vi "Blink_SDK_example_NoODP.vi"() -> ()   [LabVIEW 2010]
uses:
  Program Files/Meadowlark Optics/Blink OverDrive Plus/SDK/Blink_C_wrapper.dll
panel:
  out "ImgData 2":u8[](array[numeric])
  in  "Wait Timer":dbl
  out "Use External Triggers":bool
  out "Wavefront Correction Path":path
  out "BoardNum":i32
  out "ImgData":u8[](array[numeric])
  # "PCIe  LabVIEWSDK"
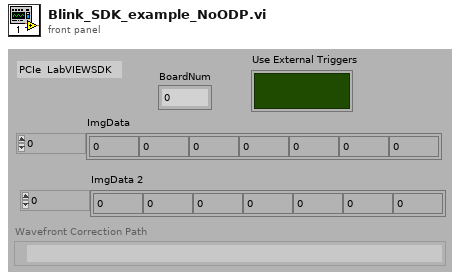
[diagram p1: front panel]
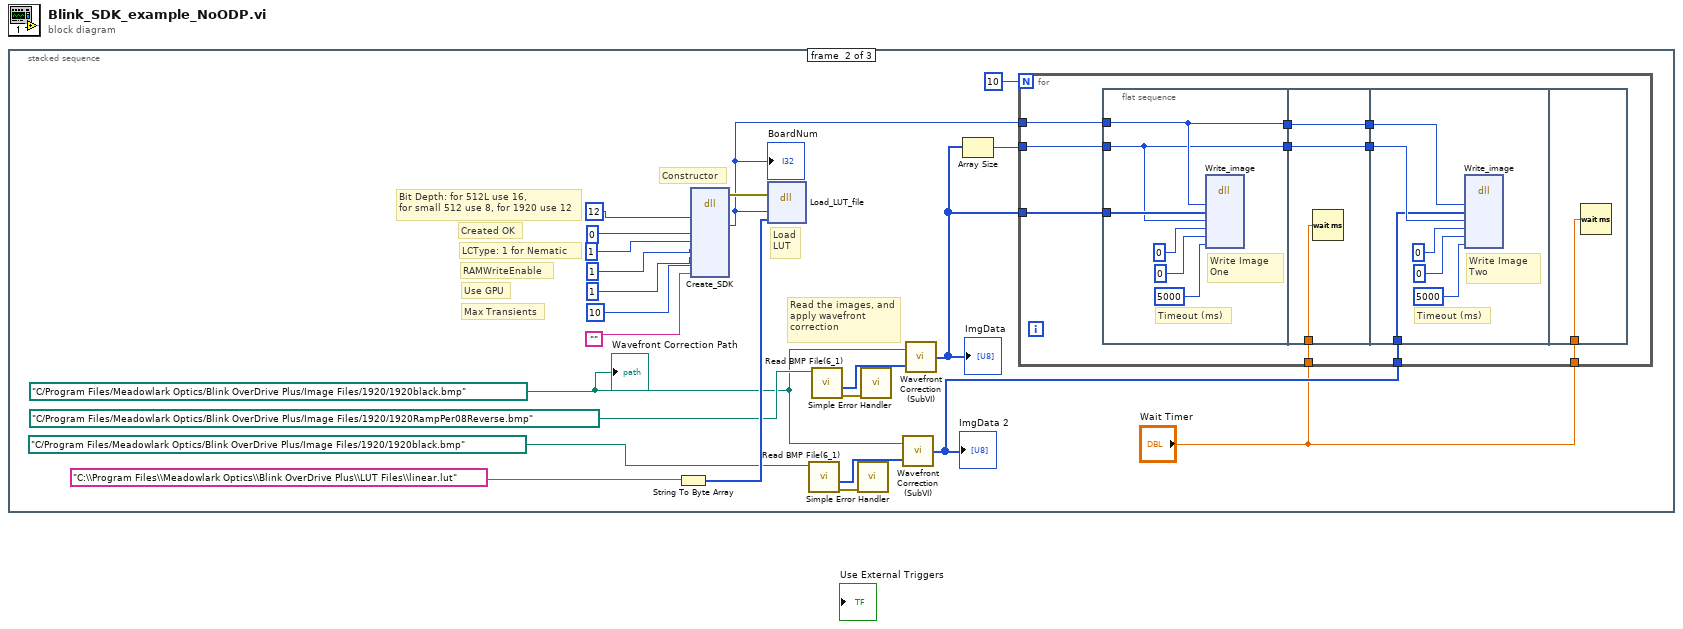
[diagram p0: block diagram]
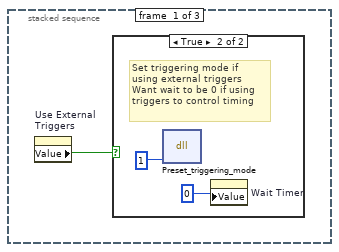
[diagram p2: hidden frame]
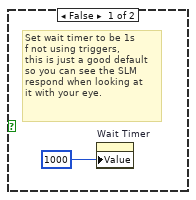
[diagram p3: hidden frame]
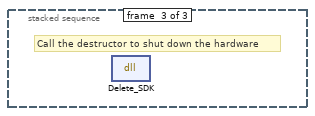
[diagram p4: hidden frame]
diagram:
  n1 = stacked-sequence {
    frame #0 {
      n2 = property on="Use External \nTriggers" class="Bool (strict)"() -> ("Value"=w1:bool)  [unwired: 2 in, 2 out]
      n3 = case shown="True" w1 {
        frame False {
          # "Set wait timer to be 1s \nf not using triggers,\nthis is just a good default \nso you can see the SLM \nrespond when looking at \nit with your eye."
          n4 = property on="Wait Timer" class="DigNum (strict)"("Value"=1000) -> ()  [unwired: 2 in, 2 out]
        }
        frame True {
          # "Set triggering mode if \nusing external triggers\nWant wait to be 0 if using \ntriggers to control timing"
          n5 = dll-call lib="C:/Program Files/Meadowlark Optics/Blink OverDrive Plus/SDK/Blink_C_wrapper.dll" fn="Preset_triggering_mode"("UseTrigger"=1) -> ()  [unwired: 5 in, 2 out]
          n6 = property on="Wait Timer" class="DigNum (strict)"("Value"=0) -> ()  [unwired: 2 in, 2 out]
        }
      }
    }
    frame #1 {
      w10 = path "C:/Program Files/Meadowlark Optics/Blink OverDrive Plus/Image Files/1920/1920black.bmp"
      # "Load\nLUT"
      # "Read the images, and apply wavefront\ncorrection"
      # "Created OK"
      # "Max Transients"
      # "Use GPU"
      # "RAMWriteEnable"
      # "Bit Depth: for 512L use 16, \nfor small 512 use 8, for 1920 use 12"
      # "LCType: 1 for Nematic"
      # "Constructor"
      n7 = String To Byte Array(string="C:\\Program Files\\Meadowlark Optics\\Blink OverDrive Plus\\LUT Files\\linear.lut") -> (unsigned byte array=w21:u8[])
      n8 = dll-call lib="C:/Program Files/Meadowlark Optics/Blink OverDrive Plus/SDK/Blink_C_wrapper.dll" fn="Create_SDK"("SLM_bit_depth"=12, "constructed_ok"=0, "is_nematic_type"=1, "RAM_write_enable"=1, "use_GPU_if_available"=1, "max_transient_frames"=10, "static_regional_lut_file"="") -> (error out=w22:errorcluster, "n_boards_found"=w6:u64)  [unwired: 12 in, 1 out]
      "BoardNum" <- w6
      n9 = dll-call lib="C:/Program Files/Meadowlark Optics/Blink OverDrive Plus/SDK/Blink_C_wrapper.dll" fn="Load_LUT_file"(error in=w22, "Board"=w6, "LUTPath"=w21) -> ()  [unwired: 5 in, 2 out]
      n10 = call <vilib>:"Read BMP File(6_1).vi"("path to BMP file"=path "C:/Program Files/Meadowlark Optics/Blink OverDrive Plus/Image Files/1920/1920black.bmp") -> ("error out"=w17:errorcluster, "flattened image data"=w18:u8[])  [unwired: 5 in, 4 out]
      n11 = call <vilib>:"Read BMP File(6_1).vi"("path to BMP file"=path "C:/Program Files/Meadowlark Optics/Blink OverDrive Plus/Image Files/1920/1920RampPer08Reverse.bmp") -> ("error out"=w19:errorcluster, "flattened image data"=w20:u8[])  [unwired: 5 in, 4 out]
      n12 = call <vilib>:"Simple Error Handler.vi"("error in (no error)"=w17) -> ()  [unwired: 4 in, 5 out]
      n13 = call <vilib>:"Simple Error Handler.vi"("error in (no error)"=w19) -> ()  [unwired: 4 in, 5 out]
      n14 = call "Wavefront Correction (SubVI).vi"("Source Image Array"=w18, "Correction Path"=w10) -> ("Corrected Image Array"=w11:u8[])
      "ImgData 2" <- w11
      n15 = call "Wavefront Correction (SubVI).vi"("Source Image Array"=w20, "Correction Path"=w10) -> ("Corrected Image Array"=w13:u8[])
      "ImgData" <- w13
      n16 = Array Size(array=w13) -> (size(s)=w12:i32)
      n17 = for {
        N: 10 -> [_]
        tunnel: w6 -> [w37]
        tunnel: w13 -> [w36]
        tunnel: w12 -> [w35]
        tunnel: w11 -> [w34]
        tunnel: "Wait Timer" -> [w29]
        tunnel: "Wait Timer" -> [w28]
        n18 = flat-sequence {
          tunnel: w37 -> [w39]
          tunnel: w36 -> [w40]
          tunnel: w35 -> [w38]
          tunnel: [w39] -> w33
          tunnel: [w38] -> w31
          tunnel: w33 -> [w46]
          tunnel: [w46] -> w32
          tunnel: w31 -> [w45]
          tunnel: [w45] -> w30
          tunnel: w29 -> [w44]
          tunnel: w32 -> [w49]
          tunnel: w30 -> [w48]
          tunnel: w34 -> [w47]
          tunnel: w28 -> [w53]
          frame #0 {
            # "Timeout (ms)"
            # "Write Image \nOne"
            n19 = dll-call lib="C:/Program Files/Meadowlark Optics/Blink OverDrive Plus/SDK/Blink_C_wrapper.dll" fn="Write_image"("board"=w39, "Image"=w40, "ImageSize"=w38, "WaitForTrigger"=0, "ExternalPulse"=0, "timeout"=5000) -> ()  [unwired: 10 in, 2 out]
          }
          frame #1 {
            n20 = Wait (ms)(milliseconds to wait=w44) -> ()  [unwired: 1 out]
          }
          frame #2 {
            # "Timeout (ms)"
            # "Write Image \nTwo"
            n21 = dll-call lib="C:/Program Files/Meadowlark Optics/Blink OverDrive Plus/SDK/Blink_C_wrapper.dll" fn="Write_image"("board"=w49, "Image"=w47, "ImageSize"=w48, "WaitForTrigger"=0, "ExternalPulse"=0, "timeout"=5000) -> ()  [unwired: 10 in, 2 out]
          }
          frame #3 {
            n22 = Wait (ms)(milliseconds to wait=w53) -> ()  [unwired: 1 out]
          }
        }
      }
      "Wavefront Correction Path" <- w10
    }
    frame #2 {
      # "Call the destructor to shut down the hardware"
      n23 = dll-call lib="C:/Program Files/Meadowlark Optics/Blink OverDrive Plus/SDK/Blink_C_wrapper.dll" fn="Delete_SDK"() -> ()  [unwired: 4 in, 2 out]
    }
  }
